vi "Periodic Tasks.vi"(8 "error in":errorcluster) -> ()   [LabVIEW 2017]
doc: "This VI runs in parallel to other robot code. It can contain as many user-defined periodic loops as you need. These can carry out PID or other sorts of timed response."
uses:
  <vilib>/Rock Robotics/WPI/Joystick/WPI_JoystickDeviceEnum.ctl
  <vilib>/Rock Robotics/WPI/Ultrasonic/WPI_SonarMB1010AnalogDeviceRef.ctl
  <vilib>/Rock Robotics/WPI/AnalogChannel/WPI_AnalogChannelDevRef.ctl
  <vilib>/Rock Robotics/SystemInterfaces/AI/FPGA_AIChannel.ctl
  <vilib>/Rock Robotics/WPI/ThirdParty/Sensors/ADIS16448 IMU/ADI_IMU_ADIS16448_IMUDevRef.ctl
  <vilib>/Rock Robotics/SystemInterfaces/spilib/spi_bus.ctl
  <vilib>/Rock Robotics/WPI/Utilities/WPI_GetSetVariantRefNum.vi
  <vilib>/Rock Robotics/WPI/Ultrasonic/WPI_SonarMB1010AnalogRefNum Registry Get.vi
  Robot Global Data.vi
  <vilib>/Rock Robotics/WPI/Ultrasonic/WPI_SonarMB1010AnalogGetRange.vi
  <vilib>/Rock Robotics/WPI/ThirdParty/Sensors/ADIS16448 IMU/ADIS16448_IMU.lvlib
panel:
  out "Current Faults":bool[](array[boolean])
  out "Battery Voltage Fault":bool
  out "Temperature Fault":bool
  out "Hardware Fault":bool
  out "IMU Angles Out":T1
  out "Z Angle":dbl
  out "Sonar Distance":dbl
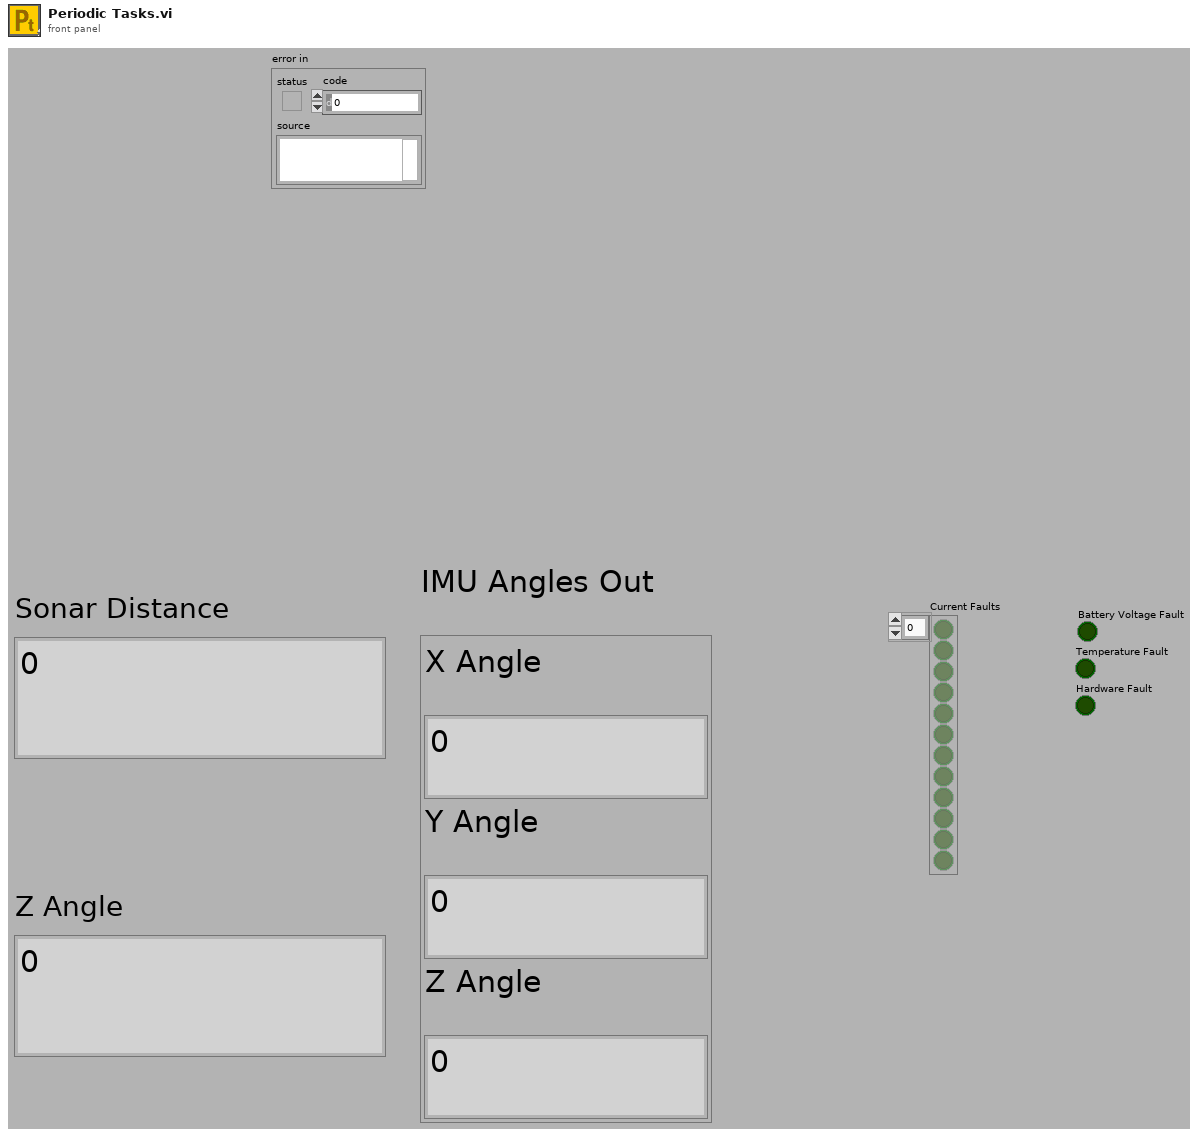
[diagram p1: front panel]
types:
  T1 = cluster{"X Angle":dbl, "Y Angle":dbl, "Z Angle":dbl}
  T2 = typedef "WPI_JoystickDeviceEnum.ctl" = enum16{"USB 0", "USB 1", "USB 2", "USB 3", "USB 4", "USB 5"}
  T3 = typedef "WPI_SonarMB1010AnalogDeviceRef.ctl" = cluster{"AIDeviceRef":T4, "Scaling factor (V/in)":dbl, "Average Bits":u8}
  T4 = typedef "WPI_AnalogChannelDevRef.ctl" = cluster{"DevStatus":errorcluster, "Analog Channel":T5}
  T5 = typedef "FPGA_AIChannel.ctl" = enum8{"AI 0", "AI 1", "AI 2", "AI 3", "AI MXP 0", "AI MXP 1", "AI MXP 2", "AI MXP 3", "Invalid"}
  T6 = typedef "ADIS16448_IMU.lvlib/ADI_IMU_ADIS16448_IMUDevRef.ctl" = cluster{"DevStatus":errorcluster, "Handle":i32, "SPI Bus":T7, "Device Found":bool, "Device Ready":bool, "Yaw Axis":enum16{"X", "Y", "Z"}, "AHRS Algorithm":enum16{"Complementary", "Madgwick"}, "Serial":u16, "Lot ID 2":u16, "Lot ID 1":u16, "Bytes Per Sample":u16, "Calibrate On Open?":bool}
  T7 = typedef "spi_bus.ctl" = enum16{"SPI On-Board, CS0", "SPI On-Board, CS1", "SPI On-Board, CS2", "SPI On-Board, CS3", "SPI MXP", "Invalid"}
  T8 = cluster{"Joystick 0":cluster{"Joystick 0":T2}, "Joystick 1":cluster{"Joystick 1":T2}, "Sonar":T3, "ADI IMU":T6}
  T9 = typedef "WPI_JoystickDevRef.ctl" = cluster{"Device":T2}
  T10 = typedef "WPI_DriverStationRobotMode2.ctl" = enum16{"Autonomous Disabled", "Autonomous Enabled", "Teleop Disabled", "Teleop Enabled", "Disconnected", "Finish", "Test Disabled", "Test Enabled", "Emergency Stopped"}
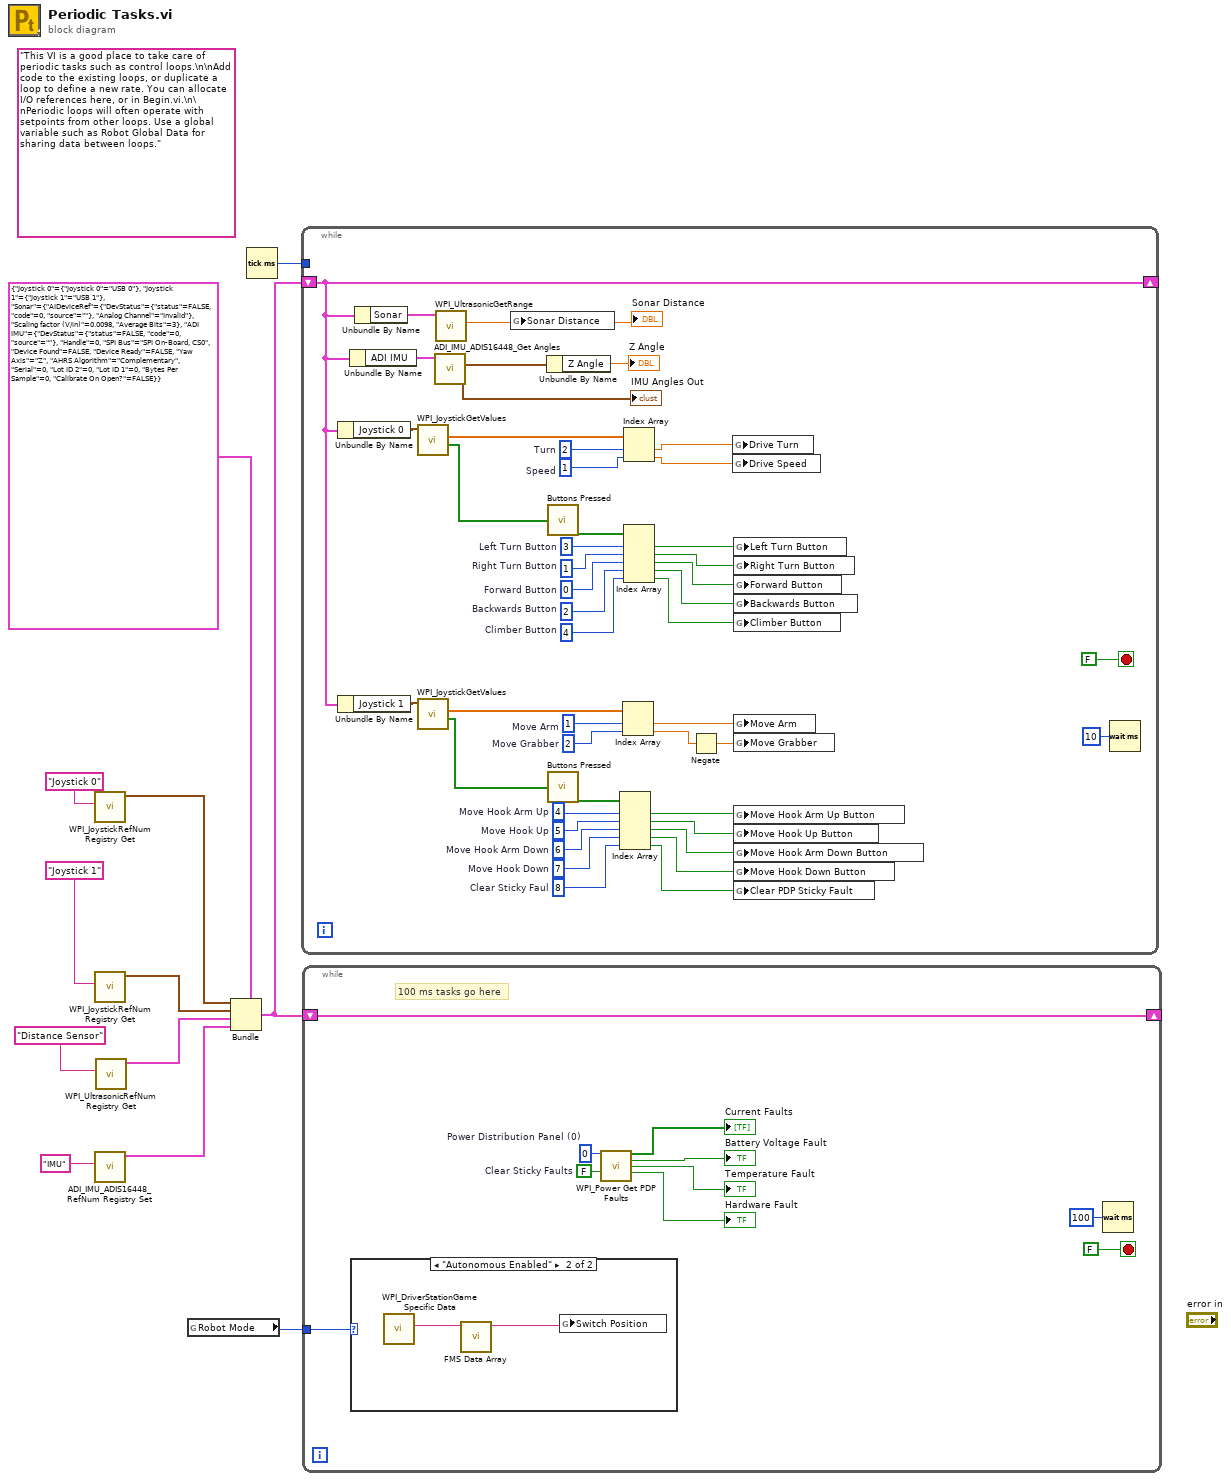
[diagram p0: block diagram]
diagram:
  (unwired) "This VI is a good place to take care of periodic tasks such as control loops.\n\nAdd code to the existing loops, or duplicate a loop to define a new rate. You can allocate I/O references here, or in Begin.vi.\n\nPeriodic loops will often operate with setpoints from other loops. Use a global variable such as Robot Global Data for sharing data between loops."
  n1 = call <vilib>:"WPI_JoystickRefNum Registry Get.vi"("refnum name"="Joystick 0") -> ("JoystickDevRef"=w9:T9)  [unwired: 1 in, 9 out]
  n2 = call <vilib>:"WPI_JoystickRefNum Registry Get.vi"("refnum name"="Joystick 1") -> ("JoystickDevRef"=w8:T9)  [unwired: 1 in, 9 out]
  n3 = call <vilib>:"ADI_IMU_ADIS16448_RefNum Registry Set.vi"("refnum name"="IMU") -> ("ADI IMU DevRef"=w2:T6)  [unwired: 9 in, 1 out]
  n4 = call-poly <vilib>:"WPI_UltrasonicRefNum Registry Get.vi"("refnum name"="Distance Sensor") -> ("SonarMB1010AnalogDevRef"=w3:T3)  [unwired: 9 in, 1 out]
  n5 = global read "Robot Global Data.vi" "Robot Mode"() -> (w1:T10)
  n6 = Bundle(cluster=T8 {"Joystick 0"={"Joystick 0"=enum."USB 0"}, "Joystick 1"={"Joystick 1"=enum."USB 1"}, "Sonar"={"AIDeviceRef"={"DevStatus"={"status"=FALSE, "code"=0, "source"=""}, "Analog Channel"=enum."Invalid"}, "Scaling factor (V/in)"=0.0098, "Average Bits"=3}, "ADI IMU"={"DevStatus"={"status"=FALSE, "code"=0, "source"=""}, "Handle"=0, "SPI Bus"=enum."SPI On-Board, CS0", "Device Found"=FALSE, "Device Ready"=FALSE, "Yaw Axis"=enum."Z", "AHRS Algorithm"=enum."Complementary", "Serial"=0, "Lot ID 2"=0, "Lot ID 1"=0, "Bytes Per Sample"=0, "Calibrate On Open?"=FALSE}}, "Joystick 0"=w9, "Joystick 1"=w8, "Sonar"=w3, "ADI IMU"=w2) -> (w7:T8)
  n7 = Tick Count (ms)() -> (millisecond timer value=w11:u32)
  n8 = while {
    shift-right: [w40] -> _
    shift-left: w7 -> [w40]
    tunnel: w11 -> [_]
    stop <- FALSE stop-if-true
    w14 = i8 4  # Climber Button
    w23 = 6  # Move Hook Arm Down
    w24 = 4  # Move Hook Arm Up
    w30 = i8 2  # Backwards Button
    w31 = i8 0  # Forward Button
    w22 = 7  # Move Hook Down
    w32 = 5  # Move Hook Up
    w27 = 2  # Move Grabber
    w28 = 1  # Move Arm
    w38 = 1  # Speed
    w39 = 2  # Turn
    w17 = i8 8  # Clear Sticky Faul
    w48 = i8 1  # Right Turn Button
    w49 = i8 3  # Left Turn Button
    n9 = Unbundle By Name(w40) -> ("Joystick 0"=w45:cluster{"Joystick 0":T2})
    n10 = Unbundle By Name(w40) -> ("Joystick 1"=w44:cluster{"Joystick 1":T2})
    n11 = Unbundle By Name(w40) -> ("ADI IMU"=w46:T6)
    n12 = Unbundle By Name(w40) -> ("Sonar"=w47:T3)
    n13 = call <vilib>:"WPI_JoystickGetValues.vi"("JoystickDevRef"=w45) -> ("Buttons"=w51:bool[], "Axes"=w52:dbl[])  [unwired: 6 in, 3 out]
    n14 = call <vilib>:"WPI_JoystickGetValues.vi"("JoystickDevRef"=w44) -> ("Buttons"=w42:bool[], "Axes"=w41:dbl[])  [unwired: 6 in, 3 out]
    n15 = call <vilib>:"ADI_IMU_ADIS16448_Get Angles.vi"("ADI IMU DevRef"=w46) -> ("IMU Angles Out"=w54:T1)  [unwired: 7 in, 3 out]
    "IMU Angles Out" <- w54
    n16 = call-poly <vilib>:"WPI_UltrasonicGetRange.vi"("SonarMB1010AnalogDevRef"=w47) -> ("Distance"=w55:dbl)  [unwired: 8 in, 2 out]
    "Sonar Distance" <- w55
    n17 = global write "Robot Global Data.vi" "Sonar Distance"(w55) -> ()
    n18 = Unbundle By Name(w54) -> ("Z Angle"=→"Z Angle":dbl)
    n19 = call "Buttons Pressed.vi"("Button Values"=w51) -> ("Button Presses"=w50:bool[])
    n20 = call "Buttons Pressed.vi"("Button Values"=w42) -> ("Button Presses"=w43:bool[])
    n21 = Index Array(array=w43, index #1=w24, index #2=w32, index #3=w23, index #4=w22, index #5=w17) -> (element #1=w21:bool, element #2=w20:bool, element #3=w19:bool, element #4=w18:bool, element #5=w16:bool)
    n22 = Index Array(array=w41, index #1=w28, index #2=w27) -> (element #1=w26:dbl, element #2=w25:dbl)
    n23 = Index Array(array=w52, index #1=w39, index #2=w38) -> (element #1=w37:dbl, element #2=w36:dbl)
    n24 = Index Array(array=w50, index #1=w49, index #2=w48, index #3=w31, index #4=w30, index #5=w14) -> (element #1=w35:bool, element #2=w34:bool, element #3=w29:bool, element #4=w15:bool, element #5=w13:bool)
    n25 = Negate(x=w25) -> (-x=w33:dbl)
    n26 = global write "Robot Global Data.vi" "Drive Turn"(w37) -> ()
    n27 = global write "Robot Global Data.vi" "Drive Speed"(w36) -> ()
    n28 = global write "Robot Global Data.vi" "Left Turn Button"(w35) -> ()
    n29 = global write "Robot Global Data.vi" "Right Turn Button"(w34) -> ()
    n30 = global write "Robot Global Data.vi" "Forward Button"(w29) -> ()
    n31 = global write "Robot Global Data.vi" "Backwards Button"(w15) -> ()
    n32 = global write "Robot Global Data.vi" "Climber Button"(w13) -> ()
    n33 = global write "Robot Global Data.vi" "Move Arm"(w26) -> ()
    n34 = global write "Robot Global Data.vi" "Move Grabber"(w33) -> ()
    n35 = global write "Robot Global Data.vi" "Move Hook Arm Up Button"(w21) -> ()
    n36 = global write "Robot Global Data.vi" "Move Hook Up Button"(w20) -> ()
    n37 = global write "Robot Global Data.vi" "Move Hook Arm Down Button"(w19) -> ()
    n38 = global write "Robot Global Data.vi" "Move Hook Down Button"(w18) -> ()
    n39 = global write "Robot Global Data.vi" "Clear PDP Sticky Fault"(w16) -> ()
    n40 = Wait (ms)(milliseconds to wait=u32 10) -> ()  [unwired: 1 out]
  }
  n41 = while {
    shift-right: [w65] -> _
    shift-left: w7 -> [w65]
    tunnel: w1 -> [w58]
    stop <- FALSE stop-if-true
    w63 = FALSE  # Clear Sticky Faults
    w64 = u8 0  # Power Distribution Panel (0)
    # "100 ms tasks go here"
    n42 = case shown="\"Autonomous Enabled\"" w58 {
      frame Default {
      }
      frame "Autonomous Enabled" {
        n43 = call <vilib>:"WPI_DriverStationGame Specific Data.vi"() -> ("Game Specific Data"=w69:string)  [unwired: 11 in]
        n44 = call "FMS Data Array.vi"("Game Data"=w69) -> ("Switch"=w68:string)  [unwired: 8 in, 2 out]
        n45 = global write "Robot Global Data.vi" "Switch Position"(w68) -> ()
      }
    }
    n46 = call <vilib>:"WPI_Power Get PDP Faults.vi"("Power Distribution Panel (0)"=w64, "Clear Sticky Faults"=w63) -> ("Current Faults"=→"Current Faults":bool[], "Battery Voltage Fault"=→"Battery Voltage Fault":bool, "Temperature Fault"=→"Temperature Fault":bool, "Hardware Fault"=→"Hardware Fault":bool)  [unwired: 9 in, 1 out]
    n47 = Wait (ms)(milliseconds to wait=u32 100) -> ()  [unwired: 1 out]
  }
